vi "Convert DC RectifierListData to Arrays.vi"(8 "error in (no error)":errorcluster, 11 "MulticolumnListbox in":refnum<vi>) -> (0 "error out":errorcluster, 2 "Right Amps":dbl[](array[numeric]), 3 "Left Amps":dbl[](array[numeric]), 4 "Right Amp Min":dbl[](array[numeric]), 5 "Left AmpMins":dbl[](array[numeric]))   [LabVIEW 2019]
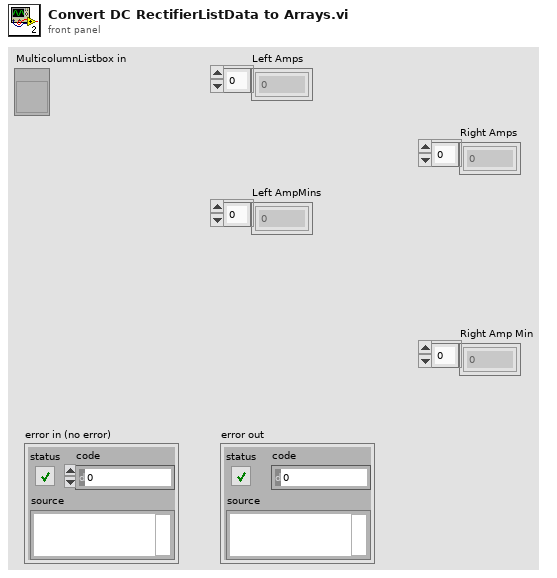
[diagram p1: front panel]
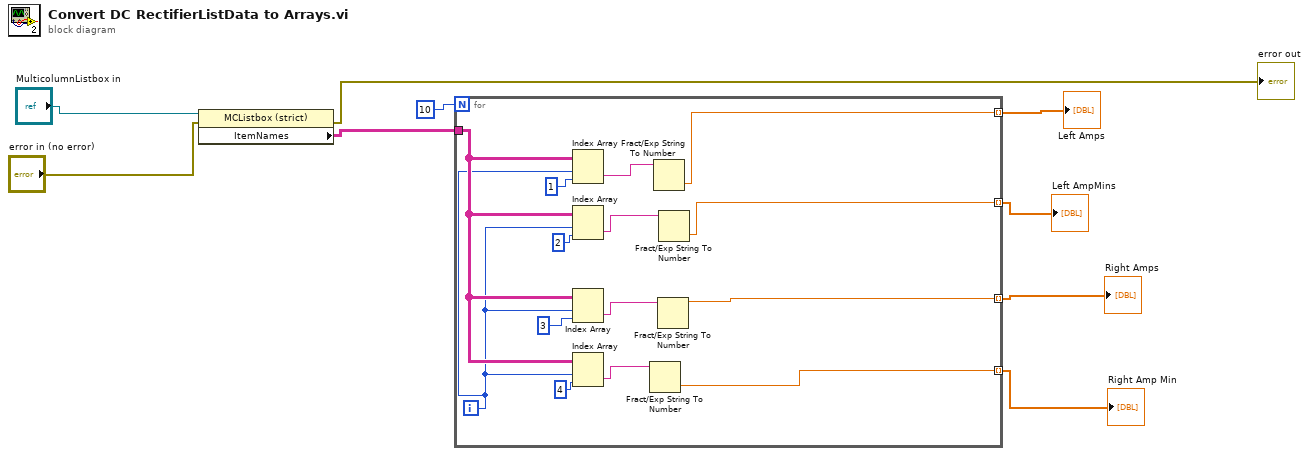
[diagram p0: block diagram]
diagram:
  n1 = property class="MCListbox (strict)"(reference="MulticolumnListbox in", error in="error in (no error)") -> (error out=→"error out":errorcluster, "ItemNames"=w8:string[][])  [unwired: 1 out]
  n2 = for {
    N: 10 -> [_]
    tunnel: w8 -> [w18]
    tunnel: [w14] -> w4 mode=indexing
    tunnel: [w11] -> w5 mode=indexing
    tunnel: [w13] -> w6 mode=indexing
    tunnel: [w10] -> w7 mode=indexing
    i -> [w12]
    n3 = Index Array(array=w18, index (row)=w12, index (col)=1 ("disabled index (col)")) -> (element=w22:string)
    n4 = Index Array(array=w18, index (row)=w12, index (col)=2 ("disabled index (col)")) -> (element=w17:string)
    n5 = Index Array(array=w18, index (row)=w12, index (col)=3 ("disabled index (col)")) -> (element=w16:string)
    n6 = Index Array(array=w18, index (row)=w12, index (col)=4 ("disabled index (col)")) -> (element=w15:string)
    n7 = Fract/Exp String To Number(string=w15) -> (number=w10:dbl)  [unwired: 3 in, 1 out]
    n8 = Fract/Exp String To Number(string=w22) -> (number=w14:dbl)  [unwired: 3 in, 1 out]
    n9 = Fract/Exp String To Number(string=w16) -> (number=w13:dbl)  [unwired: 3 in, 1 out]
    n10 = Fract/Exp String To Number(string=w17) -> (number=w11:dbl)  [unwired: 3 in, 1 out]
  }
  "Right Amp Min" <- w7
  "Right Amps" <- w6
  "Left AmpMins" <- w5
  "Left Amps" <- w4
